vi "Softsign.vi"(2 "Z":dbl) -> (0 "Softsign(Z)":dbl)   [LabVIEW 2020]
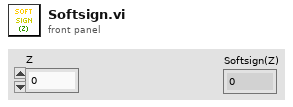
[diagram p1: front panel]
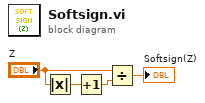
[diagram p0: block diagram]
diagram:
  n1 = Absolute Value(x="Z") -> (abs(x)=w3:dbl)
  n2 = Increment(x=w3) -> (x+1=w2:dbl)
  n3 = Divide(x="Z", y=w2) -> (x/y=→"Softsign(Z)":dbl)
